vi "Document_AddContent.vi"(8 "error in (no error)":errorcluster, 10 "Content":refnum<k24>, 11 "ooWriter in":refnum<class "ooWriter.lvclass">) -> (0 "error out":errorcluster, 3 "ooWriter out":refnum<class "ooWriter.lvclass">)   [LabVIEW 2009, in "ooWriter.lvclass"]
uses:
  ooWriter.lvclass
  C:/Projets/LAVAG/OpenOfficeRGT/AODL/DLLs/AODL.dll
  ooWriter.lvclass/ooWriter.ctl
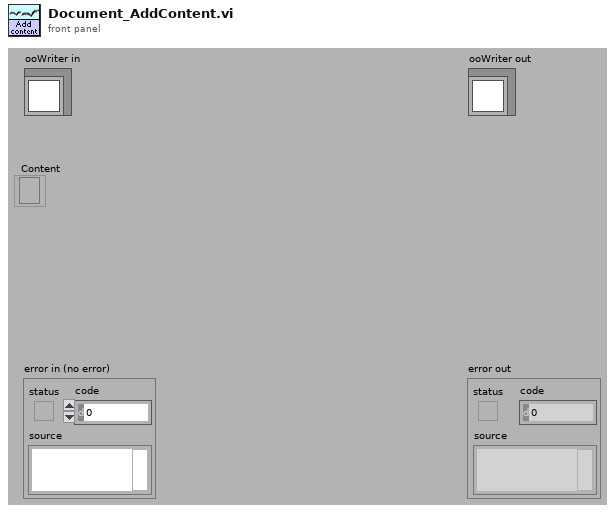
[diagram p1: front panel]
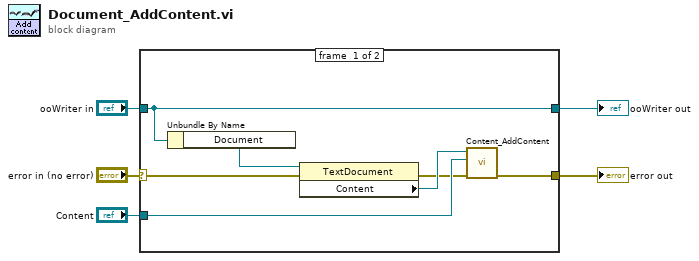
[diagram p0: block diagram]
diagram:
  n1 = case shown="No Error" "error in (no error)" {
    selector: "error in (no error)" -> [w7 w14]
    tunnel: [w6 w14] -> w5
    tunnel: [w11 w13] -> w3
    tunnel: "ooWriter in" -> [w11 w13]
    tunnel: "Content" -> [w9 _]
    frame #0 {
      n2 = Unbundle By Name(w11) -> ("Document"=w12:refnum<k24>)
      n3 = property class="TextDocument"(reference=w12, error in=w7) -> (error out=w8:errorcluster, "Content"=w10:refnum<k24>)  [unwired: 1 out]
      n4 = call "Content_AddContent.vi"("error in"=w8, "Content"=w9, "ContentCollection"=w10) -> ("error out"=w6:errorcluster)  [unwired: 7 in, 1 out]
    }
    frame #1 {
    }
  }
  "error out" <- w5
  "ooWriter out" <- w3
